vi "Add Recipe.vi"(8 "error in (no error)":errorcluster, 11 "Master in":refnum<class "Master.lvclass">) -> (0 "error out":errorcluster, 3 "Master out":refnum<class "Master.lvclass">)   [LabVIEW 2014, in "Master.lvclass"]
uses:
  Master/Master.lvclass
panel:
  in  "Cancel":bool
  in  "Add":bool
  in  "Control Panel":T1 {"Unit" items=["mm", "inch"]}
  # "RPS"
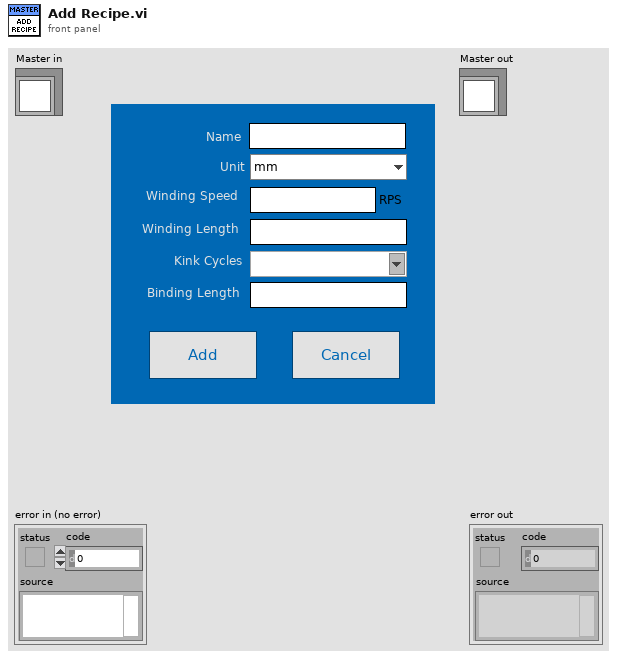
[diagram p1: front panel]
types:
  T1 = cluster{"Name":string, "Unit":u16, "Winding Speed":string, "Winding Length":string, "Kink Cycles":string, "Binding Length":string}
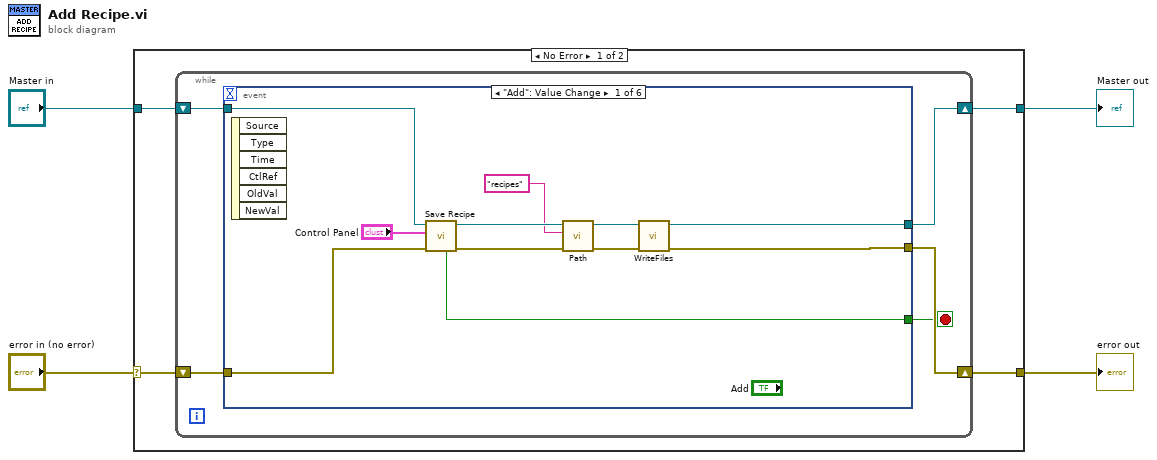
[diagram p0: block diagram]
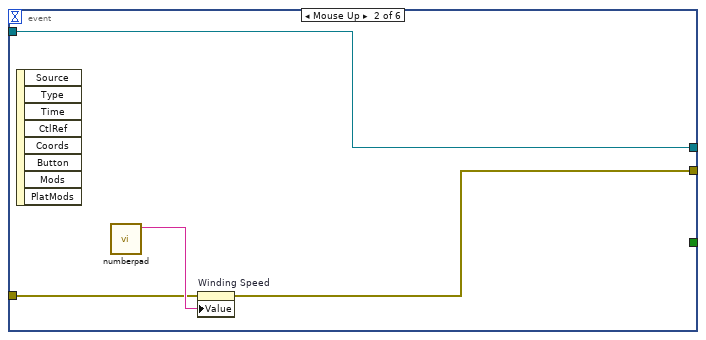
[diagram p2: hidden frame]
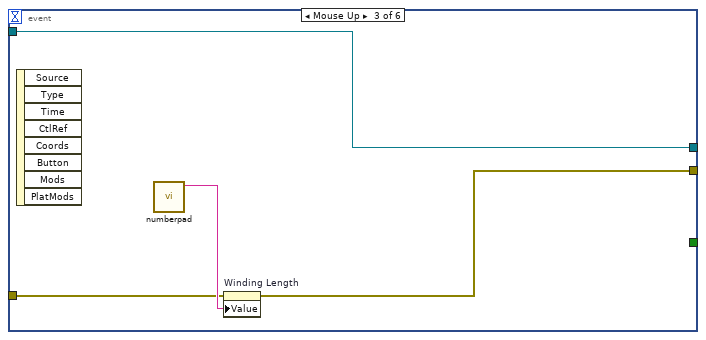
[diagram p3: hidden frame]
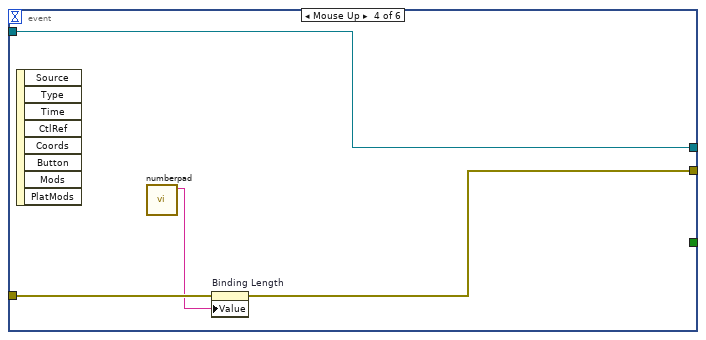
[diagram p4: hidden frame]
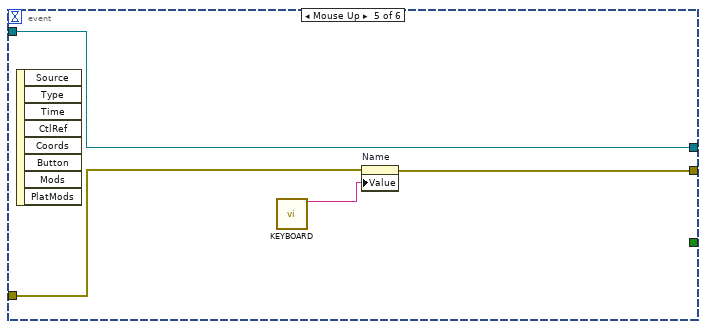
[diagram p5: hidden frame]
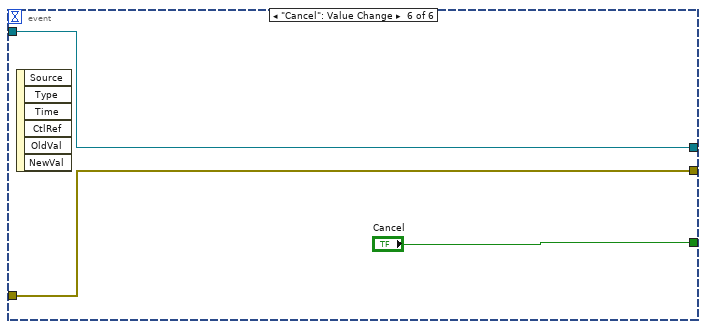
[diagram p6: hidden frame]
diagram:
  n1 = case shown="No Error" "error in (no error)" {
    selector: "error in (no error)" -> [w7 w45]
    tunnel: [w5 w45] -> w3
    tunnel: [w6 w44] -> w1
    tunnel: "Master in" -> [w8 w44]
    frame No Error {
      n2 = while {
        shift-right: [w12] -> w6
        shift-left: w8 -> [w13]
        shift-right: [w10] -> w5
        shift-left: w7 -> [w11]
        stop <- w9 stop-if-true
        n3 = event shown="[0] \"Add\": Value Change" {
          selector: _ -> [_ _ _ _ _ _]
          dyn-events: _ -> [_ _ _ _ _ _]
          timeout: _ -> [_ _ _ _ _ _]
          tunnel: w13 -> [w24 w25 w29 w36 w40 w42]
          tunnel: [w15 w25 w29 w36 w40 w42] -> w12
          tunnel: w11 -> [w23 w27 w30 w34 w38 w41]
          tunnel: [w16 w26 w31 w35 w39 w41] -> w10
          tunnel: [w17 _ _ _ _ "Cancel"] -> w9
          event "Add": Value Change {
            n4 = event-data() -> ()  [unwired: 1 in, 6 out]
            n5 = call-dynamic "Save Recipe.vi"("error in (no error)"=w23, "Control Panel"="Control Panel", "Master in"=w24) -> ("error out"=w20:errorcluster, "Master out"=w22:refnum<class "Master.lvclass">, "Save"=w17:bool)  [unwired: 6 in]
            n6 = call-dynamic "Path.vi"("error in (no error)"=w20, "pathname"="recipes", "Master in"=w22) -> ("error out"=w18:errorcluster, "Master out"=w19:refnum<class "Master.lvclass">)  [unwired: 7 in]
            n7 = call-dynamic "WriteFiles.vi"("error in (no error)"=w18, "Master in"=w19) -> ("error out"=w16:errorcluster, "Master out"=w15:refnum<class "Master.lvclass">)  [unwired: 8 in]
          }
          event "Control Panel.Winding Speed": Mouse Up {
            n8 = event-data() -> ()  [unwired: 1 in, 8 out]
            n9 = call "numberpad.vi"() -> ("String"=w28:string)  [unwired: 11 in]
            n10 = property on="Winding Speed" class="Str"(error in=w27, "Value"=w28) -> (error out=w26:errorcluster)  [unwired: 1 in, 1 out]
          }
          event "Control Panel.Winding Length": Mouse Up {
            n11 = event-data() -> ()  [unwired: 1 in, 8 out]
            n12 = call "numberpad.vi"() -> ("String"=w32:string)  [unwired: 11 in]
            n13 = property on="Winding Length" class="Str"(error in=w30, "Value"=w32) -> (error out=w31:errorcluster)  [unwired: 1 in, 1 out]
          }
          event "Control Panel.Binding Length": Mouse Up {
            n14 = event-data() -> ()  [unwired: 1 in, 8 out]
            n15 = call "numberpad.vi"() -> ("String"=w33:string)  [unwired: 11 in]
            n16 = property on="Binding Length" class="Str"(error in=w34, "Value"=w33) -> (error out=w35:errorcluster)  [unwired: 1 in, 1 out]
          }
          event "Control Panel.Name": Mouse Up {
            n17 = event-data() -> ()  [unwired: 1 in, 8 out]
            n18 = call "KEYBOARD.vi"() -> ("String"=w37:string)  [unwired: 15 in]
            n19 = property on="Name" class="Str"(error in=w38, "Value"=w37) -> (error out=w39:errorcluster)  [unwired: 1 in, 1 out]
          }
          event "Cancel": Value Change {
            n20 = event-data() -> ()  [unwired: 1 in, 6 out]
          }
        }
      }
    }
    frame Error {
    }
  }
  "error out" <- w3
  "Master out" <- w1
